vi "Initialize Server State.vi"(8 "error in":errorcluster, 10 "Initial State":T1, 11 "gRPC server in":refnum<class "Servicer.lvclass">) -> (0 "error out":errorcluster, 3 "gRPC server out":refnum<class "Servicer.lvclass">)   [LabVIEW 2019, in "gRPC-servicer.lvlib" / "Servicer.lvclass"]
uses:
  Servicer.lvclass
  typeDefs/Server State Data.ctl
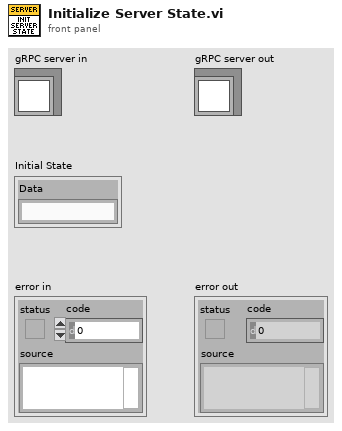
[diagram p1: front panel]
types:
  T1 = typedef "gRPC-servicer.lvlib/Servicer.lvclass/Server State Data.ctl" = cluster{"Data":string}
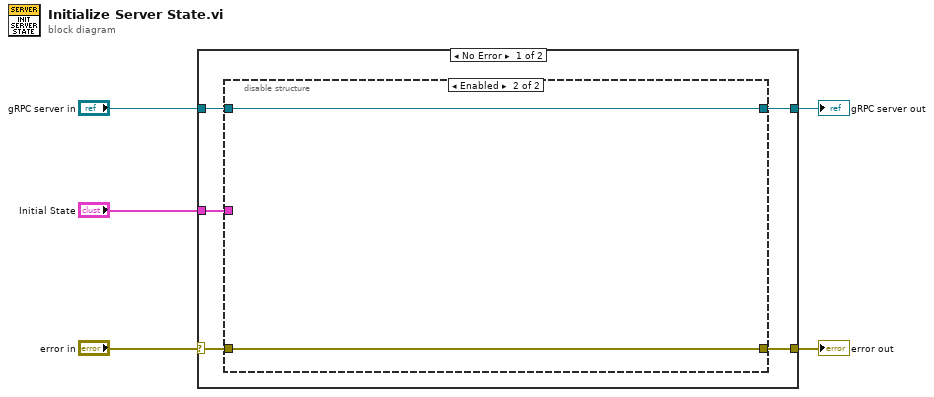
[diagram p0: block diagram]
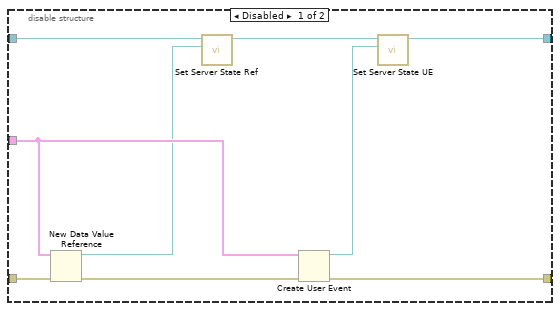
[diagram p2: hidden frame]
diagram:
  n1 = case shown="No Error" "error in" {
    selector: "error in" -> [w10 w23]
    tunnel: [w9 w23] -> w4
    tunnel: [w6 w22] -> w2
    tunnel: "gRPC server in" -> [w7 w22]
    tunnel: "Initial State" -> [w8 _]
    frame No Error {
      n2 = disable-structure shown="Enabled" {
        disable-tunnel: w10 -> [w18 w21]
        disable-tunnel: [w17 w21] -> w9
        disable-tunnel: w8 -> [w16 _]
        disable-tunnel: w7 -> [w15 w20]
        disable-tunnel: [w12 w20] -> w6
        frame Disabled {
          n3 = New Data Value Reference(data value=w16, error in=w18) -> (data value reference=w14:refnum<data-value>, error out=w19:errorcluster)
          n4 = call "Set Server State Ref.vi"("Server Internal State Ref"=w14, "gRPC server in"=w15) -> ("gRPC server out"=w13:refnum<class "Servicer.lvclass">)  [unwired: 9 in]
          n5 = Create User Event(user event datatype=w16, error in=w19) -> (user event=w11:refnum<user-event>, error out=w17:errorcluster)
          n6 = call "Set Server State UE.vi"("Server State UE"=w11, "gRPC server in"=w13) -> ("gRPC server out"=w12:refnum<class "Servicer.lvclass">)  [unwired: 9 in]
        }
        frame Enabled {
        }
      }
    }
    frame Error {
    }
  }
  "error out" <- w4
  "gRPC server out" <- w2
